vi "AddOrChangeLine(SubVI).vi"(8 "error in (no error)":errorcluster, 11 "String in":string) -> (0 "error out":errorcluster, 1 "String Array Out":string[](array[string]), 2 "Enum":enum16{"Default", "Change", "Add"}(ring), 3 "String out":string)   [LabVIEW 2018]
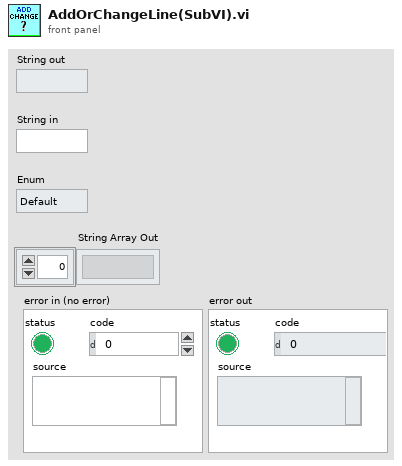
[diagram p1: front panel]
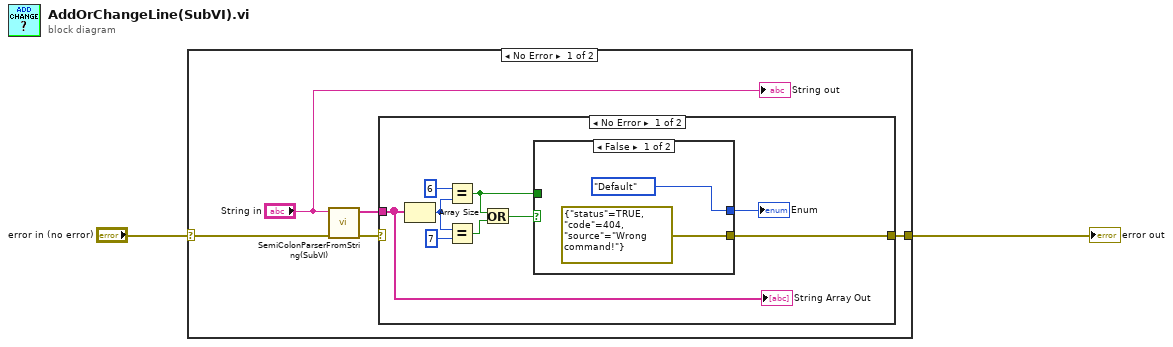
[diagram p0: block diagram]
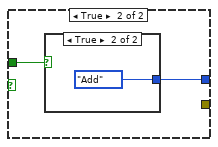
[diagram p2: hidden frame]
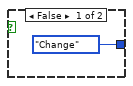
[diagram p3: hidden frame]
diagram:
  n1 = case shown="No Error" "error in (no error)" {
    selector: "error in (no error)" -> [w7 w24]
    tunnel: [w4 w24] -> w1
    frame No Error {
      n2 = call "SemiColonParserFromString(SubVI).vi"("Error In"=w7, "String In"="String in") -> ("Error Out"=w5:errorcluster, "String Array Out"=w6:string[])  [unwired: 8 in]
      n3 = case shown="No Error" w5 {
        selector: w5 -> [_ w23]
        tunnel: w6 -> [w8 _]
        tunnel: [w9 w23] -> w4
        frame No Error {
          n4 = Array Size(array=w8) -> (size(s)=w15:i32)
          n5 = Equal?(x=6, y=w15) -> (x = y?=w11:bool)
          n6 = Equal?(x=w15, y=7) -> (x = y?=w13:bool)
          n7 = Or(x=w11, y=w13) -> (x .or. y?=w12:bool)
          n8 = case shown="False" w12 {
            tunnel: w11 -> [_ w20]
            tunnel: [enum16{"Default", "Change", "Add"}."Default" ("Enum") w19] -> w10
            tunnel: [errorcluster {"status"=TRUE, "code"=404, "source"="Wrong command!"} ("error IO") _] -> w9
            frame False {
            }
            frame True {
              n9 = case shown="True" w20 {
                tunnel: [enum16{"Default", "Change", "Add"}."Change" ("Enum") enum16{"Default", "Change", "Add"}."Add" ("Enum")] -> w19
                frame False {
                }
                frame True {
                }
              }
            }
          }
          "Enum" <- w10
          "String Array Out" <- w8
        }
        frame Error {
        }
      }
      "String out" <- "String in"
    }
    frame Error {
    }
  }
  "error out" <- w1
